vi "MultiOpto_1.2_Begin.vi"() -> (0 "Текущий Образец №":string, 1 "NI Scope Status":bool, 2 "Ophir 1 Status":bool, 3 "Ophir 2 Status":bool, 4 "DC Power 1 Status":bool, 6 "DC Power 2 Status":bool, 8 "NI DMM 1 Status":bool, 10 "NI DMM 2 Status":bool, 11 "Stepper Motor Status":bool, 12 "NI DMM 3 option return":enum32{"Ampermeter button", "Ohmmeter button"}(ring), 13 "NI DMM 2 option return":enum32{"Ampermeter button", "Ohmmeter button"}(ring), 14 "NI DMM 1 option return":enum32{"Ampermeter button", "Ohmmeter button"}(ring), 15 "NI DMM 3 Status":bool)   [LabVIEW 2018]
panel:
  in  "DC Power 1":bool
  in  "DC Power 2":bool
  in  "OK Button":bool
  in  "Stepper Motor":bool
  in  "NI DMM 3 option":enum32{"Ampermeter button", "Ohmmeter button"}(radio)
  in  "NI DMM 3":bool
  in  "NI DMM 2 option":enum32{"Ampermeter button", "Ohmmeter button"}(radio)
  in  "NI DMM 1 option":enum32{"Ampermeter button", "Ohmmeter button"}(radio)
  in  "Ophir 2":bool
  in  "NI DMM 2":bool
  out "Boolean 4":bool
  out "Boolean 3":bool
  in  "Ophir 1":bool
  in  "NI DMM 1":bool
  in  "NI Scope":bool
  in  "Образец №":string
  out "Boolean":bool
  out "Boolean 2":bool
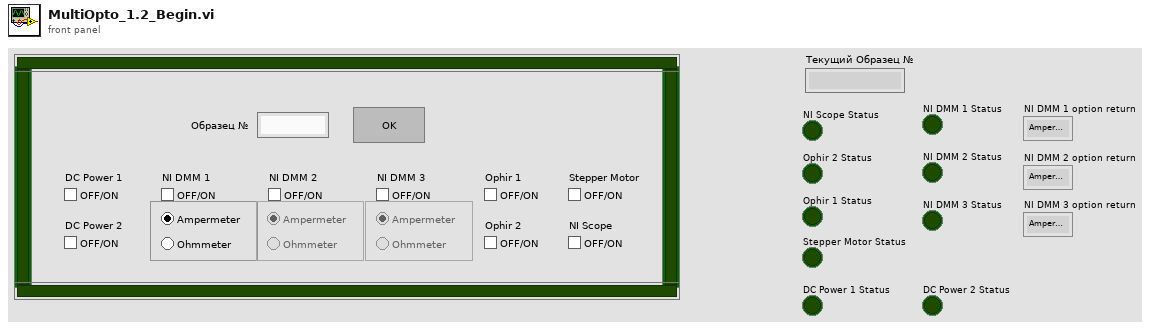
[diagram p1: front panel]
types:
  T1 = enum8{"Enabled", "Disabled", "Disabled and Grayed Out"}
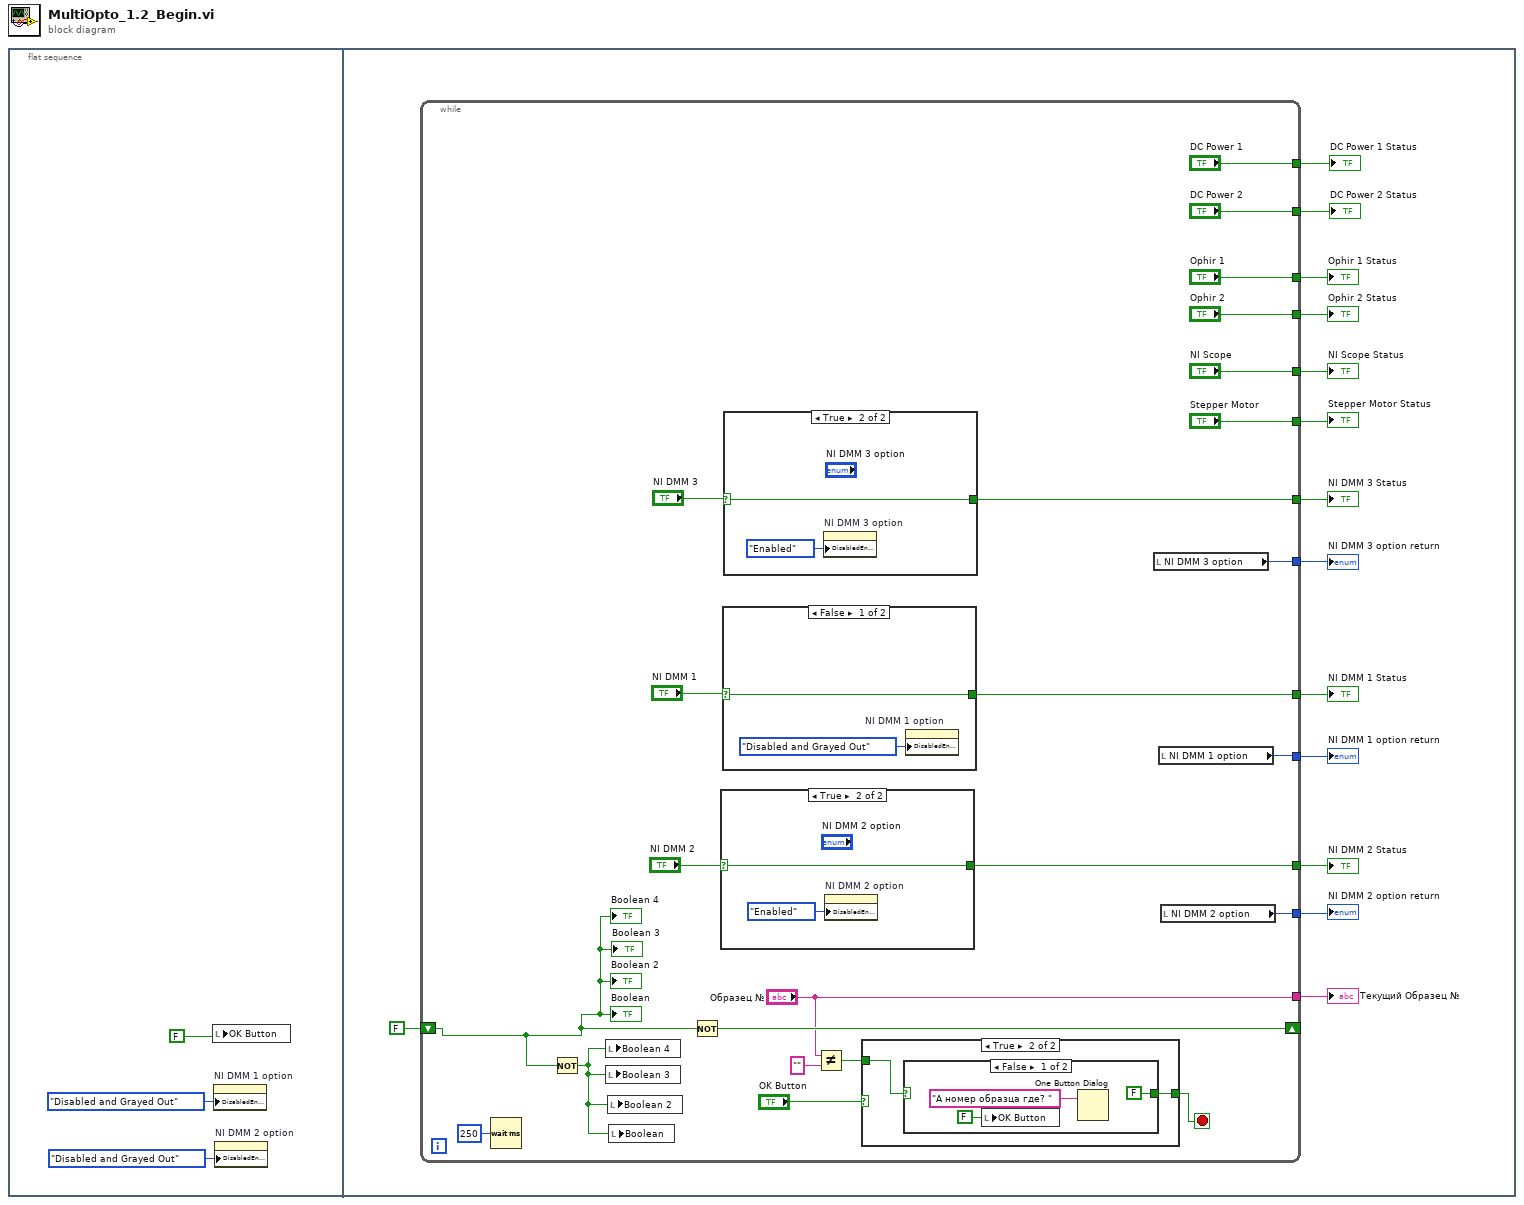
[diagram p0: block diagram]
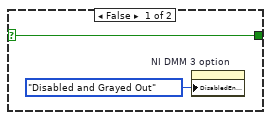
[diagram p4: hidden frame]
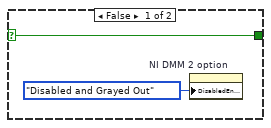
[diagram p5: hidden frame]
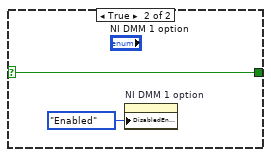
[diagram p6: hidden frame]
diagram:
  n1 = flat-sequence {
    frame #0 {
      n2 = local write "OK Button"(FALSE ("Ввел!")) -> ()
      n3 = property on="NI DMM 1 option" class="RadioBtnsControl (strict)"("DisabledEnum"=T1."Disabled and Grayed Out" ("Disabled")) -> ()  [unwired: 2 in, 2 out]
      n4 = property on="NI DMM 2 option" class="RadioBtnsControl (strict)"("DisabledEnum"=T1."Disabled and Grayed Out" ("Disabled")) -> ()  [unwired: 2 in, 2 out]
    }
    frame #1 {
      n5 = while {
        tunnel: ["Образец №"] -> w17
        shift-right: [w40] -> _
        shift-left: FALSE -> [w39]
        tunnel: ["NI Scope"] -> w15
        tunnel: [w32] -> w14
        tunnel: ["Ophir 1"] -> w13
        tunnel: [w31] -> w12
        tunnel: ["Ophir 2"] -> w11
        tunnel: [w30] -> w10
        tunnel: [w29] -> w9
        tunnel: [w27] -> w8
        tunnel: [w26] -> w7
        tunnel: ["Stepper Motor"] -> w6
        tunnel: ["DC Power 1"] -> w5
        tunnel: ["DC Power 2"] -> w4
        stop <- w22 stop-if-true
        n6 = Wait (ms)(milliseconds to wait=u32 250) -> ()  [unwired: 1 out]
        n7 = Not(x=w39) -> (.not. x?=w38:bool)
        n8 = local write "Boolean 4"(w38) -> ()
        n9 = local write "Boolean 3"(w38) -> ()
        n10 = local write "Boolean 2"(w38) -> ()
        n11 = local write "Boolean"(w38) -> ()
        n12 = Not(x=w39) -> (.not. x?=w40:bool)
        n13 = case shown="True" "NI DMM 2" {
          selector: "NI DMM 2" -> [w53 w56]
          tunnel: [w53 w56] -> w31
          frame False {
            n14 = property on="NI DMM 2 option" class="RadioBtnsControl (strict)"("DisabledEnum"=T1."Disabled and Grayed Out" ("Disabled")) -> ()  [unwired: 2 in, 2 out]
          }
          frame True {
            n15 = property on="NI DMM 2 option" class="RadioBtnsControl (strict)"("DisabledEnum"=T1."Enabled" ("Disabled")) -> ()  [unwired: 2 in, 2 out]
          }
        }
        n16 = case shown="False" "NI DMM 1" {
          selector: "NI DMM 1" -> [w57 w60]
          tunnel: [w57 w60] -> w32
          frame False {
            n17 = property on="NI DMM 1 option" class="RadioBtnsControl (strict)"("DisabledEnum"=T1."Disabled and Grayed Out" ("Disabled")) -> ()  [unwired: 2 in, 2 out]
          }
          frame True {
            n18 = property on="NI DMM 1 option" class="RadioBtnsControl (strict)"("DisabledEnum"=T1."Enabled" ("Disabled")) -> ()  [unwired: 2 in, 2 out]
          }
        }
        n19 = case shown="True" "NI DMM 3" {
          selector: "NI DMM 3" -> [w49 w52]
          tunnel: [w49 w52] -> w27
          frame False {
            n20 = property on="NI DMM 3 option" class="RadioBtnsControl (strict)"("DisabledEnum"=T1."Disabled and Grayed Out" ("Disabled")) -> ()  [unwired: 2 in, 2 out]
          }
          frame True {
            n21 = property on="NI DMM 3 option" class="RadioBtnsControl (strict)"("DisabledEnum"=T1."Enabled" ("Disabled")) -> ()  [unwired: 2 in, 2 out]
          }
        }
        n22 = Not Equal?(x="Образец №", y="") -> (x != y?=w23:bool)
        n23 = case shown="True" "OK Button" {
          selector: "OK Button" -> [w42 _]
          tunnel: w23 -> [_ w44]
          tunnel: [w42 w43] -> w22
          frame False {
          }
          frame True {
            n24 = case shown="False" w44 {
              selector: w44 -> [_ w48]
              tunnel: [FALSE w48] -> w43
              frame False {
                n25 = local write "OK Button"(FALSE ("OK Button")) -> ()
                n26 = One Button Dialog(message="А номер образца где? ") -> ()  [unwired: 1 in, 1 out]
              }
              frame True {
              }
            }
          }
        }
        n27 = local read "NI DMM 3 option"() -> (w26:enum32{"Ampermeter button", "Ohmmeter button"})
        n28 = local read "NI DMM 1 option"() -> (w30:enum32{"Ampermeter button", "Ohmmeter button"})
        n29 = local read "NI DMM 2 option"() -> (w29:enum32{"Ampermeter button", "Ohmmeter button"})
        "Boolean" <- w39
        "Boolean 2" <- w39
        "Boolean 3" <- w39
        "Boolean 4" <- w39
      }
      "Текущий Образец №" <- w17
      "NI Scope Status" <- w15
      "NI DMM 1 Status" <- w14
      "Ophir 1 Status" <- w13
      "NI DMM 2 Status" <- w12
      "Ophir 2 Status" <- w11
      "NI DMM 2 option return" <- w9
      "NI DMM 1 option return" <- w10
      "NI DMM 3 Status" <- w8
      "NI DMM 3 option return" <- w7
      "Stepper Motor Status" <- w6
      "DC Power 1 Status" <- w5
      "DC Power 2 Status" <- w4
    }
  }
